vi "VISATCP组合选择发送.vi"(0 "IP":string, 1 "数据发送通道":enum16{"TCP", "VISA"}(ring), 2 "命令":string(combo), 5 "PORT":string, 7 "VISA resource name":refnum<visa-resource-name> caption="VISA资源名称", 9 "baud rate":u32=115200 caption="波特率(115200)", 11 "error in (no error)":errorcluster caption="错误输入（无错误）", 12 "写入缓冲区":string) -> (4 "连接ID":refnum<k5>, 6 "VISA resource name 2":refnum<visa-resource-name>, 13 "读取缓冲区":string, 15 "错误输出":errorcluster)   [LabVIEW 2016, in "数据传输系统.lvlib"]
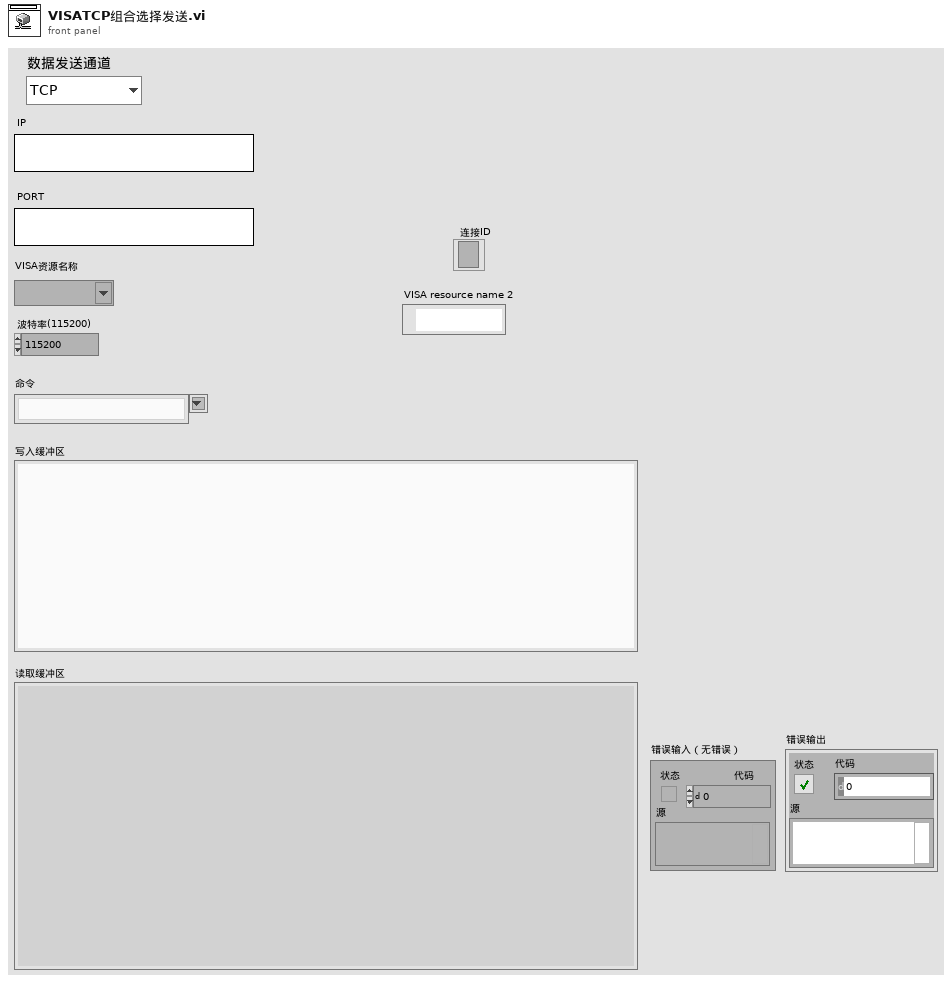
[diagram p1: front panel]
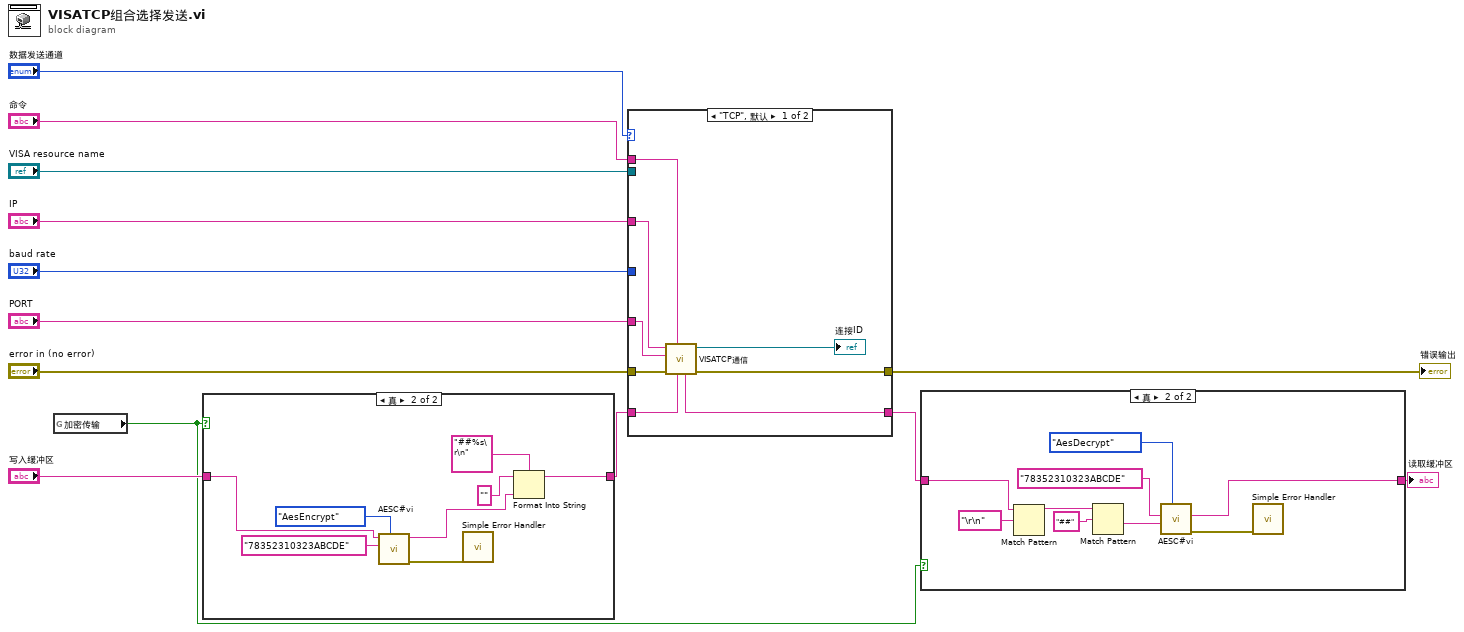
[diagram p0: block diagram]
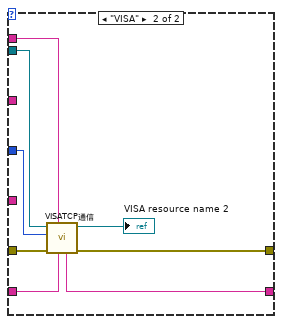
[diagram p4: hidden frame]
diagram:
  n1 = global read "断电保存全局.vi" "加密传输"() -> (w3:bool)
  n2 = case shown="真" w3 {
    tunnel: "写入缓冲区" -> [w14 w22]
    tunnel: [w14 w21] -> w4
    frame False {
    }
    frame True {
      n3 = call "AESC#vi.vi"("枚举"=enum16{"AesEncrypt", "AesDecrypt"}."AesEncrypt", "key"="78352310323ABCDE", "plainText"=w22) -> ("错误输出"=w15:errorcluster, "AESEncrypt"=w16:string)  [unwired: 6 in, 1 out]
      n4 = call <vilib>:"Simple Error Handler.vi"("error in (no error)"=w15) -> ()  [unwired: 4 in, 5 out]
      n5 = Format Into String(format string="##%s\r\n", initial string="" ("初始字符串"), w16) -> (resulting string=w21:string)  [unwired: 1 in, 1 out]
    }
  }
  n6 = case shown="\"TCP\", 默认" "数据发送通道" {
    tunnel: "命令" -> [w30 w34]
    tunnel: [w29 w36] -> w11
    tunnel: "error in (no error)" -> [w28 w35]
    tunnel: w4 -> [w27 w38]
    tunnel: [w26 w37] -> w2
    tunnel: "PORT" -> [w25 _]
    tunnel: "IP" -> [w24 _]
    tunnel: "baud rate" -> [_ w32]
    tunnel: "VISA resource name" -> [_ w31]
    frame "TCP", Default {
      n7 = call-poly "VISATCP通信.vi"("写入缓冲区"=w27, "命令"=w30, "error in (no error)"=w28, "PORT"=w25, "IP"=w24) -> ("错误输出"=w29:errorcluster, "连接ID"=→"连接ID":refnum<k5>, "读取缓冲区"=w26:string)  [unwired: 4 in]
    }
    frame "VISA" {
      n8 = call-poly "VISATCP通信.vi"("写入缓冲区"=w38, "命令"=w34, "error in (no error)"=w35, "baud rate (9600)"=w32, "VISA resource name"=w31) -> ("错误输出"=w36:errorcluster, "VISA resource name 2"=→"VISA resource name 2":refnum<visa-resource-name>, "读取缓冲区"=w37:string)  [unwired: 4 in]
    }
  }
  "错误输出" <- w11
  n9 = case shown="真" w3 {
    tunnel: w2 -> [w39 w47]
    tunnel: [w39 w48] -> w1
    frame False {
    }
    frame True {
      n10 = Match Pattern(string=w47, regular expression="\r\n" ("正则表达式")) -> (before substring=w42:string)  [unwired: 1 in, 3 out]
      n11 = Match Pattern(string=w42, regular expression="##" ("正则表达式")) -> (after substring=w41:string)  [unwired: 1 in, 3 out]
      n12 = call "AESC#vi.vi"("枚举"=enum16{"AesEncrypt", "AesDecrypt"}."AesDecrypt", "encryptStr"=w41, "key"="78352310323ABCDE") -> ("错误输出"=w40:errorcluster, "AESDecrypt"=w48:string)  [unwired: 6 in, 1 out]
      n13 = call <vilib>:"Simple Error Handler.vi"("error in (no error)"=w40) -> ()  [unwired: 4 in, 5 out]
    }
  }
  "读取缓冲区" <- w1
